vi "deleteCategory.vi"(8 "error in (no error)":errorcluster, 10 "Category Name":string, 11 "Database in":refnum<class "Account History.lvclass">) -> (0 "error out":errorcluster, 3 "Database out":refnum<class "Account History.lvclass">)   [LabVIEW 2018, in "Account History.lvclass"]
uses:
  Account History.lvclass
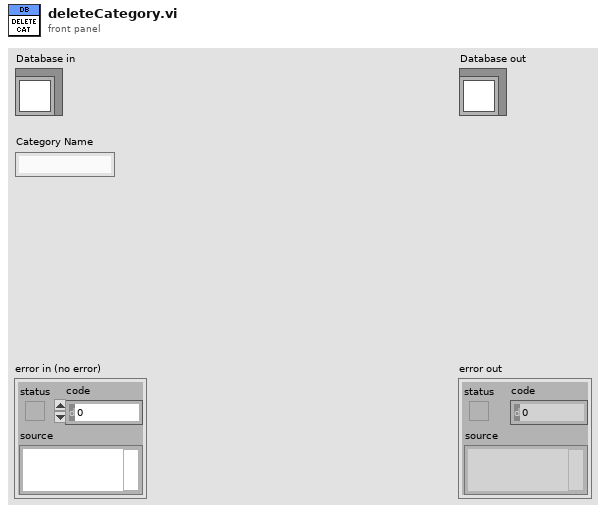
[diagram p1: front panel]
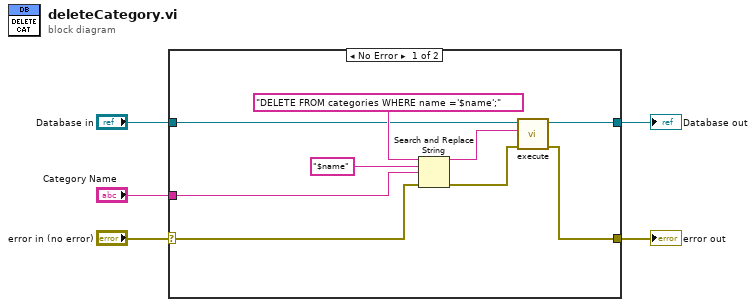
[diagram p0: block diagram]
diagram:
  n1 = case shown="No Error" "error in (no error)" {
    selector: "error in (no error)" -> [w7 w15]
    tunnel: "Database in" -> [w13 w16]
    tunnel: [w12 w16] -> w4
    tunnel: [w11 w15] -> w3
    tunnel: "Category Name" -> [w6 _]
    frame No Error {
      n2 = Search and Replace String(input string="DELETE FROM categories WHERE name ='$name';", search string="$name", replace string=w6, error in=w7) -> (result string=w10:string, error out=w9:errorcluster)  [unwired: 4 in, 2 out]
      n3 = call "execute.vi"("error in (no error)"=w9, "SQL query"=w10, "Database in"=w13) -> ("error out"=w11:errorcluster, "Database out"=w12:refnum<class "Account History.lvclass">)  [unwired: 7 in]
    }
    frame Error {
    }
  }
  "error out" <- w3
  "Database out" <- w4
